vi "GetBandBounds.vi"(8 "error in (no error)":errorcluster, 11 "Properties In":T1[](array[typedef])) -> (0 "error out":errorcluster, 1 "High":sgl, 2 "Low":sgl, 3 "Properties Out":T1[](array[typedef]))   [LabVIEW 2017, in "AnalysisHelper.lvlib"]
uses:
  <vilib>/addons/InsightCM/Utilities/Analysis/Shared/AnalysisHelper.lvlib
  <vilib>/addons/InsightCM/MessageBus/Base/controls/KeyValuePair.ctl
  <vilib>/addons/InsightCM/Utilities/PropertyHelpers/PropertyHelpers.lvlib
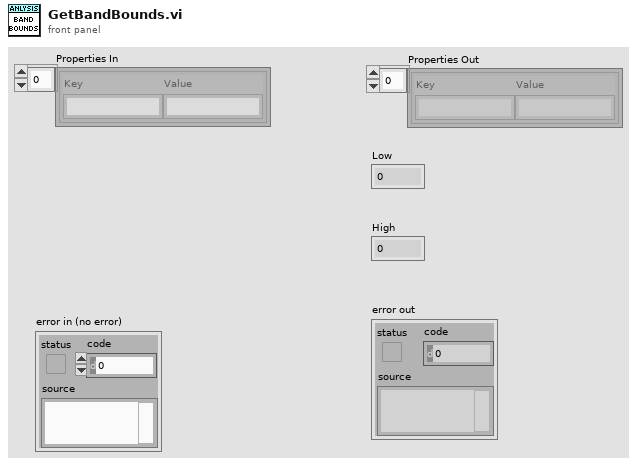
[diagram p1: front panel]
types:
  T1 = typedef "KeyValuePair.ctl" = cluster{"Key":string, "Value":string}
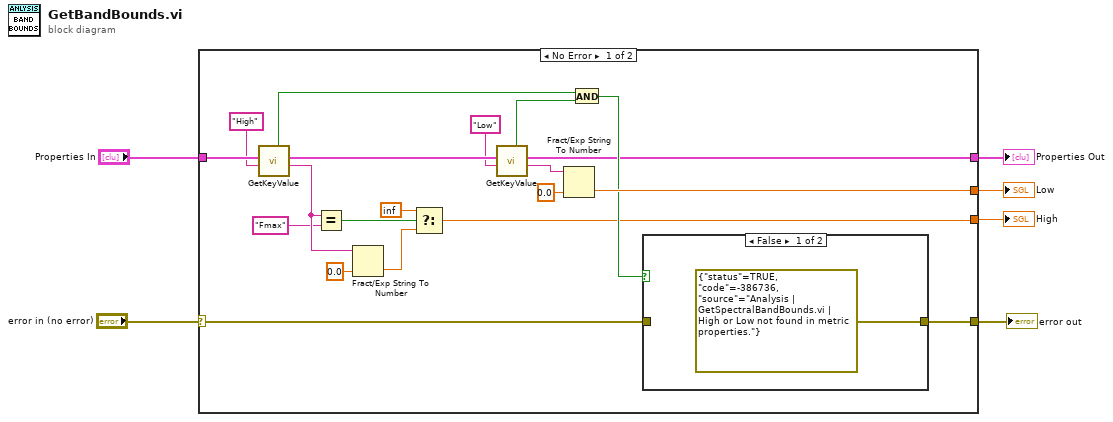
[diagram p0: block diagram]
diagram:
  n1 = case shown="No Error" "error in (no error)" {
    selector: "error in (no error)" -> [w20 w30]
    tunnel: [w19 w29] -> w6
    tunnel: [w7 _] -> w5
    tunnel: [w25 _] -> w4
    tunnel: "Properties In" -> [w18 w29]
    tunnel: [w21 w30] -> w1
    frame No Error {
      n2 = call <vilib>:"GetKeyValue.vi"("key"="High", "key value pairs"=w18) -> ("value"=w12:string, "key value pairs out"=w17:T1[], "found"=w23:bool)  [unwired: 7 in]
      n3 = Equal?(x=w12, y="Fmax") -> (x = y?=w10:bool)
      n4 = Fract/Exp String To Number(string=w12, default (0 dbl)=sgl 0.0 ("default (0 DBL)")) -> (number=w8:sgl)  [unwired: 2 in, 1 out]
      n5 = Select(t=sgl inf, s=w10, f=w8) -> (s? t:f=w7:sgl)
      n6 = call <vilib>:"GetKeyValue.vi"("key"="Low", "key value pairs"=w17) -> ("value"=w14:string, "key value pairs out"=w19:T1[], "found"=w24:bool)  [unwired: 7 in]
      n7 = Fract/Exp String To Number(string=w14, default (0 dbl)=sgl 0.0 ("default (0 DBL)")) -> (number=w25:sgl)  [unwired: 2 in, 1 out]
      n8 = And(x=w23, y=w24) -> (x .and. y?=w22:bool)
      n9 = case shown="False" w22 {
        tunnel: [errorcluster {"status"=TRUE, "code"=-386736, "source"="Analysis | GetSpectralBandBounds.vi | High or Low not found in metric properties."} ("error in") w28] -> w21
        tunnel: w20 -> [_ w28]
        frame False {
        }
        frame True {
        }
      }
    }
    frame Error {
    }
  }
  "High" <- w5
  "Low" <- w4
  "Properties Out" <- w6
  "error out" <- w1
